vi "Alarm lesen.vi"(8 "error in (no error)":errorcluster caption="Fehler (Eingang, kein Fehler)", 11 "Steuerung PNS (Eingang)":refnum<class "Steuerung PNS.lvclass">) -> (0 "error out":errorcluster caption="Fehler (Ausgang)", 2 "Alarm":T1, 3 "Steuerung PNS (Ausgang)":refnum<class "Steuerung PNS.lvclass">)   [LabVIEW 2020, in "Steuerung PNS.lvclass"]
uses:
  Steuerung PNS.lvclass
  Alarme.ctl
  Steuerung PNS.lvclass/Steuerung PNS.ctl
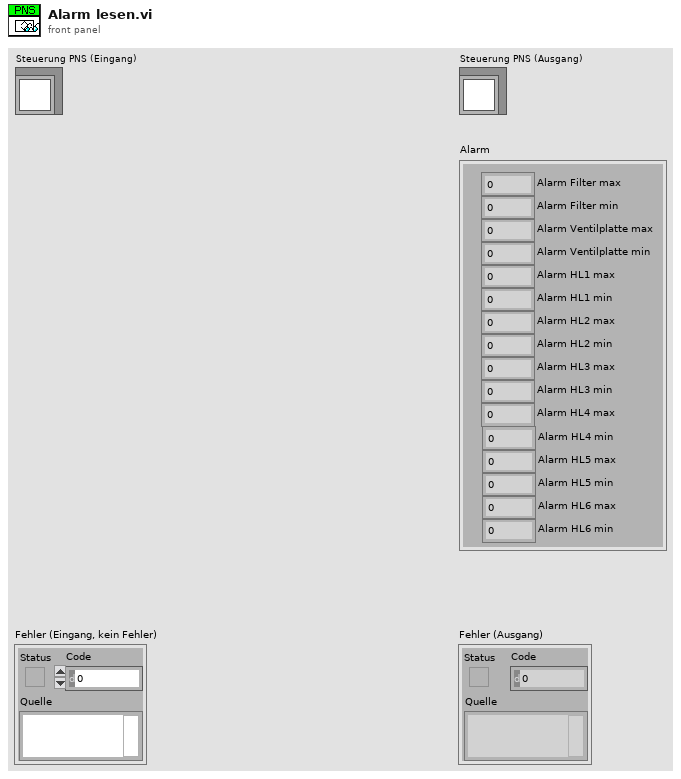
[diagram p1: front panel]
types:
  T1 = typedef "Steuerung PNS.lvclass/Alarme.ctl" = cluster{"Alarm Filter max":u16, "Alarm Filter min":u16, "Alarm Ventilplatte max":u16, "Alarm Ventilplatte min":u16, "Alarm HL1 max":u16, "Alarm HL1 min":u16, "Alarm HL2 max":u16, "Alarm HL2 min":u16, "Alarm HL3 max":u16, "Alarm HL3 min":u16, "Alarm HL4 max":u16, "Alarm HL4 min":u16, "Alarm HL5 max":u16, "Alarm HL5 min":u16, "Alarm HL6 max":u16, "Alarm HL6 min":u16}
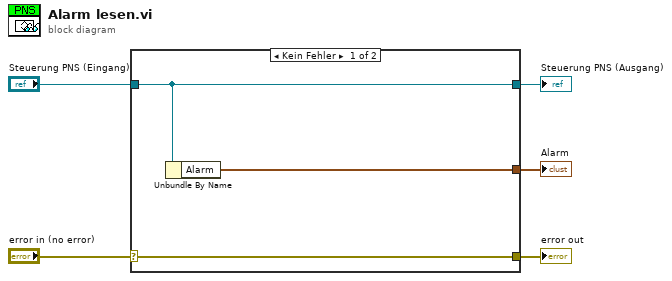
[diagram p0: block diagram]
diagram:
  n1 = case shown="Kein Fehler" "error in (no error)" {
    selector: "error in (no error)" -> [w8 w9]
    tunnel: [w8 w9] -> w4
    tunnel: [w7 w10] -> w2
    tunnel: "Steuerung PNS (Eingang)" -> [w7 w10]
    tunnel: [w6 _] -> w1
    frame No Error {
      n2 = Unbundle By Name(w7) -> ("Alarm"=w6:T1)
    }
    frame Error {
    }
  }
  "error out" <- w4
  "Steuerung PNS (Ausgang)" <- w2
  "Alarm" <- w1
